vi "Build Global Data.vi"(7 "Target":T1, 10 "Image Size":T7, 11 "Results":T2 {"Score" format="%#_3g"; "Pixels"."Box"."Bottom" format="%#_3g"; "Pixels"."Box"."Right" format="%#_3g"; "Pixels"."Box"."Top" format="%#_3g"; "Pixels"."Box"."Left" format="%#_3g"; "Normalized"."Box"."Bottom" format="%#_3g"; "Normalized"."Box"."Right" format="%#_3g"; "Normalized"."Box"."Top" format="%#_3g"; "Normalized"."Box"."Left" format="%#_3g"; "Distance (ft)" format="%#_3g"}) -> (3 "Vision Data Out":T6)   [LabVIEW 2017, in "VisionSystem.lvlib"]
uses:
  VisionSystem.lvlib
  <vilib>/Rock Robotics/WPI/Camera/WPI_CameraImageSize.ctl
  Cluster_Vision Status.ctl
  Enum_ Field Targets.ctl
  Cluster_Results.ctl
  Cluster_Targeting Data.ctl
  Cluster_SGL Point.ctl
  Cluster_UI DBL Box.ctl
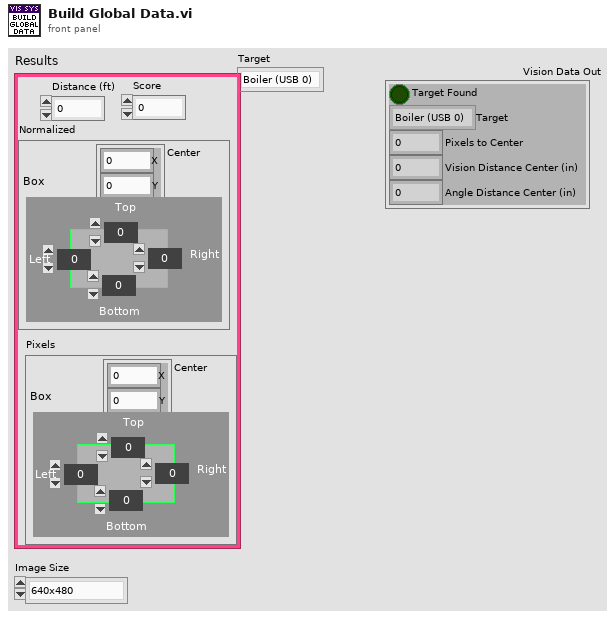
[diagram p1: front panel]
types:
  T1 = typedef "VisionSystem.lvlib/Enum_ Field Targets.ctl" = enum16{"Boiler (USB 0)", "Rope (USB 1)"}
  T2 = typedef "VisionSystem.lvlib/Cluster_Results.ctl" = cluster{"Distance (ft)":dbl, "Score":dbl, "Normalized":T3, "Pixels":T3}
  T3 = typedef "VisionSystem.lvlib/Cluster_Targeting Data.ctl" = cluster{"Center":T4, "Box":T5}
  T4 = typedef "VisionSystem.lvlib/Cluster_SGL Point.ctl" = cluster{"X":sgl, "Y":sgl}
  T5 = typedef "VisionSystem.lvlib/Cluster_UI DBL Box.ctl" = cluster{"Left":dbl, "Top":dbl, "Right":dbl, "Bottom":dbl}
  T6 = typedef "VisionSystem.lvlib/Cluster_Vision Status.ctl" = cluster{"Target Found":bool, "Target":T1, "Pixels to Center":dbl, "Vision Distance Center (in)":dbl, "Angle Distance Center (in)":dbl}
  T7 = typedef "WPI_CameraImageSize.ctl" = enum16{"640x480", "320x240", "160x120", "Custom"}
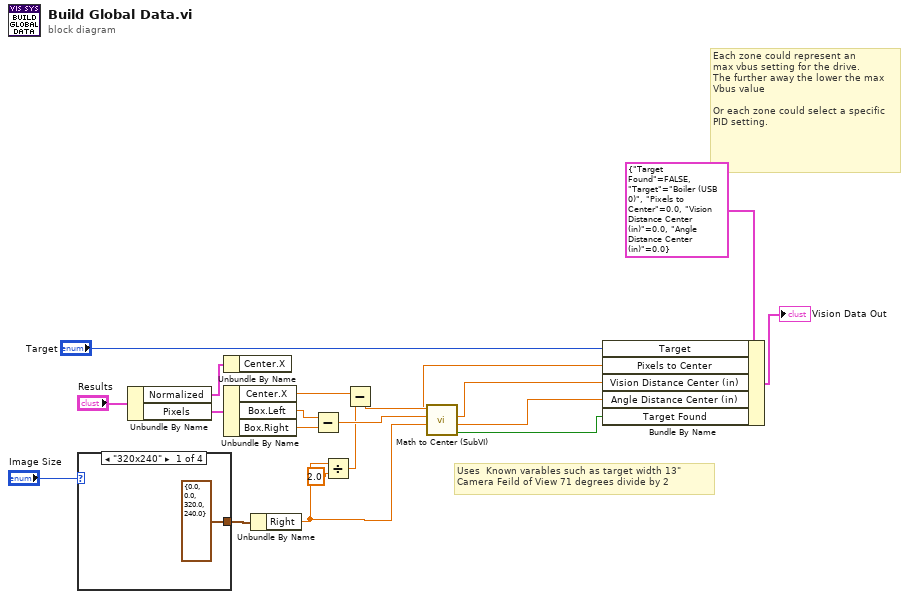
[diagram p0: block diagram]
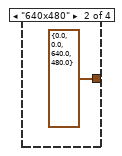
[diagram p2: hidden frame]
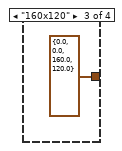
[diagram p3: hidden frame]
diagram:
  # "Uses  Known varables such as target width 13\"\nCamera Feild of View 71 degrees divide by 2"
  # "Each zone could represent an\nmax vbus setting for the drive.  \nThe further away the lower the max\nVbus value\n\nOr each zone could select a specific PID setting."
  n1 = case shown="\"320x240\"" "Image Size" {
    tunnel: [T5 {"Left"=0.0, "Top"=0.0, "Right"=320.0, "Bottom"=240.0} ("Total Box") T5 {"Left"=0.0, "Top"=0.0, "Right"=640.0, "Bottom"=480.0} ("Total Box") T5 {"Left"=0.0, "Top"=0.0, "Right"=160.0, "Bottom"=120.0} ("Total Box") _] -> w14
    frame "320x240" {
    }
    frame "640x480" {
    }
    frame "160x120" {
    }
    frame "Custom" {
    }
  }
  n2 = Unbundle By Name("Results") -> ("Normalized"=w20:T3, "Pixels"=w15:T3)
  n3 = Unbundle By Name(w20) -> ()  [unwired: 1 out]
  n4 = Unbundle By Name(w15) -> ("Center.X"=w6:sgl, "Box.Left"=w13:dbl, "Box.Right"=w12:dbl)
  n5 = Unbundle By Name(w14) -> ("Right"=w9:dbl)
  n6 = Subtract(x=w13, y=w12) -> (x-y=w11:dbl)
  n7 = Divide(x=w9, y=2.0) -> (x/y=w8:dbl)
  n8 = Subtract(x=w6, y=w8) -> (x-y=w7:dbl)
  n9 = call "Math to Center (SubVI).vi"("R Horizontal Image Resolution"=w9, "N Width Of Target (Pixels)"=w11, "Pixels To Center"=w7) -> ("Target Found Out"=w2:bool, "Degrees To Center (Degree) Out"=w1:dbl, "Distance To Target (Inches) Out"=w4:dbl, "Distance To Center (Inches) Out"=w5:dbl)  [unwired: 5 in]
  n10 = Bundle By Name(cluster=T6 {"Target Found"=FALSE, "Target"=enum."Boiler (USB 0)", "Pixels to Center"=0.0, "Vision Distance Center (in)"=0.0, "Angle Distance Center (in)"=0.0} ("Vision Data"), "Target"="Target", "Pixels to Center"=w5, "Vision Distance Center (in)"=w4, "Angle Distance Center (in)"=w1, "Target Found"=w2) -> (→"Vision Data Out":T6)
